vi "Send Receive LaunchPad.vi"(0 "VISA resource":refnum<visa-resource-name>, 5 "write buffer":string, 7 "Bytes To Read (0)":u8, 9 "Max Retries  (10)":i32=10, 11 "error in":errorcluster, 12 "Time Out (100 ms)":i32=100) -> (4 "VISA resource 2":refnum<visa-resource-name>, 6 "Read Buffer":string, 15 "error out":errorcluster)   [LabVIEW 2011]
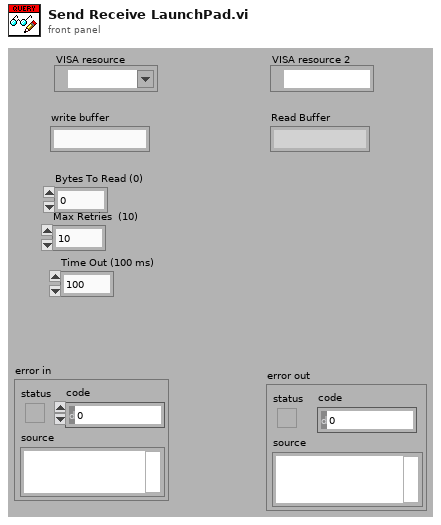
[diagram p1: front panel]
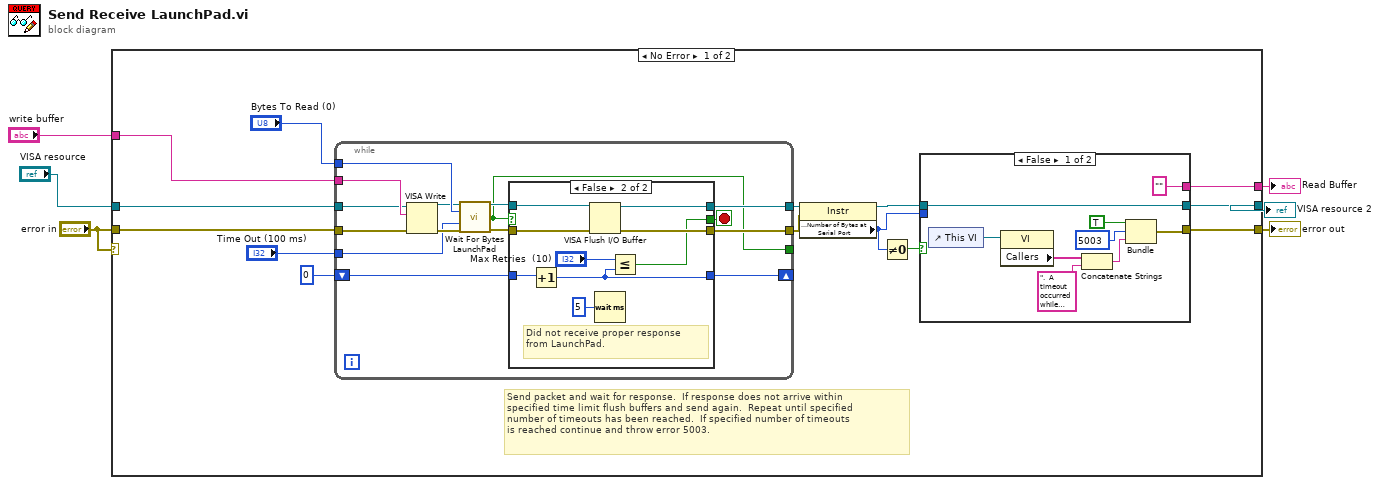
[diagram p0: block diagram]
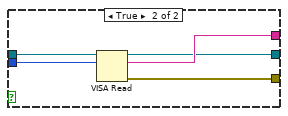
[diagram p3: hidden frame]
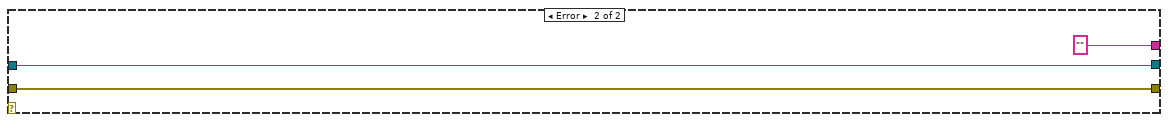
[diagram p4: hidden frame]
diagram:
  n1 = case shown="No Error" "error in" {
    tunnel: [w20 w65] -> w6
    tunnel: [w19 "" ("read buffer")] -> w5
    tunnel: "error in" -> [w14 w65]
    tunnel: "VISA resource" -> [w15 w63]
    tunnel: "write buffer" -> [w13 _]
    tunnel: [w12 w63] -> w1
    frame No Error {
      # "Send packet and wait for response.  If response does not arrive within \nspecified time limit flush buffers and send again.  Repeat until specified \nnumber of timeouts has been reached.  If specified number of timeouts\nis reached continue and throw error 5003."
      n2 = while {
        tunnel: w13 -> [w35]
        tunnel: [w29] -> w7
        tunnel: w14 -> [w34]
        tunnel: w15 -> [w33]
        tunnel: "Bytes To Read (0)" -> [w25]
        tunnel: "Time Out (100 ms)" -> [w26]
        tunnel: [w21] -> _
        shift-right: [w31] -> _
        shift-left: 0 -> [w32]
        tunnel: [w28] -> w8
        stop <- w30 stop-if-true
        n3 = VISA Write(VISA resource name=w33, write buffer=w35, error in (no error)=w34) -> (VISA resource name out=w24:refnum<visa-resource-name>, error out=w27:errorcluster)  [unwired: 1 out]
        n4 = call "Wait For Bytes LaunchPad.vi"("VISA resource"=w24, "Bytes To Read"=w25, "Time Out (100 ms)"=w26, "error in"=w27) -> ("VISA resource"=w23:refnum<visa-resource-name>, "Bytes Available?"=w21:bool, "error out"=w22:errorcluster)  [unwired: 9 in]
        n5 = case shown="False" w21 {
          selector: w21 -> [w38 _]
          tunnel: w32 -> [w39 w48]
          tunnel: [w39 w42] -> w31
          tunnel: [w38 w41] -> w30
          tunnel: w22 -> [w36 w46]
          tunnel: [w37 w45] -> w29
          tunnel: w23 -> [w37 w44]
          tunnel: [w36 w43] -> w28
          frame True {
          }
          frame False {
            # "Did not receive proper response\nfrom LaunchPad."
            n6 = Increment(x=w48) -> (x+1=w42:i32)
            n7 = VISA Flush I/O Buffer(VISA resource name=w44, error in (no error)=w46) -> (VISA resource name out=w45:refnum<visa-resource-name>, error out=w43:errorcluster)  [unwired: 1 in]
            n8 = Wait (ms)(milliseconds to wait=u32 5) -> ()  [unwired: 1 out]
            n9 = Less Or Equal?(x="Max Retries  (10)", y=w42) -> (x <= y?=w41:bool)
          }
        }
      }
      n10 = property class="Instr"(reference=w7, error in=w8) -> (reference out=w11:refnum<visa-resource-name>, "Serial Settings:Number of Bytes at Serial Port"=w9:u32)  [unwired: 1 out]
      n11 = Not Equal To 0?(x=w9) -> (x != 0?=w10:bool)
      n12 = case shown="False" w10 {
        tunnel: [w52 w62] -> w20
        tunnel: ["" ("read buffer") w61] -> w19
        tunnel: w11 -> [w57 w60]
        tunnel: [w57 w59] -> w12
        tunnel: w9 -> [_ w58]
        frame False {
          n13 = control-ref of="This VI"() -> (w53:refnum<vi>)
          n14 = property class="VI"(reference=w53) -> ("Callers"=w54:string[])  [unwired: 1 in, 2 out]
          n15 = Concatenate Strings(w54, ".  A timeout occurred while trying to read form the LaunchPAd." ("string")) -> (w51:string)
          n16 = Bundle(TRUE, "code"=5003, w51) -> (w52:cluster{bool, "code":i32, string})  [unwired: 1 in]
        }
        frame True {
          n17 = VISA Read(VISA resource name=w60, byte count=w58) -> (VISA resource name out=w59:refnum<visa-resource-name>, read buffer=w61:string, error out=w62:errorcluster)  [unwired: 1 in, 1 out]
        }
      }
    }
    frame Error {
    }
  }
  "error out" <- w6
  "Read Buffer" <- w5
  "VISA resource 2" <- w1
